vi "getStatusContainer.vi"(8 "error in (no error)":errorcluster, 11 "IComponent in":refnum<class "IComponent.lvclass">) -> (0 "error out":errorcluster, 2 "IComponentStatusContainer out":refnum<class "IComponentStatusContainer.lvclass">, 3 "IComponent out":refnum<class "IComponent.lvclass">)   [LabVIEW 2022 SP3, in "openDAQ.lvlib" / "IBaseObject.lvlib" / "IPropertyObject.lvlib" / "IComponent.lvlib" / "IComponent.lvclass"]
uses:
  <instrlib>/openDAQ/Public/Classes/IComponent/IComponent.lvclass
  C:/Program Files (x86)/National Instruments/LabVIEW 2022/instr.lib/openDAQ/Public/Classes/IBaseObject/IBaseObject.lvclass
  <instrlib>/openDAQ/Public/Classes/IComponentStatusContainer/IComponentStatusContainer.lvclass
  <instrlib>/openDAQ/Public/Classes/IBaseObject/IBaseObject.lvclass/IBaseObject.ctl
  <instrlib>/openDAQ/Public/Classes/IBaseObject/Accessor/Read reference.vi
  <instrlib>/openDAQ/Public/Classes/IBaseObject/Accessor/Write reference.vi
  <instrlib>/openDAQ/Binaries/Windows/x86/copendaq32.dll
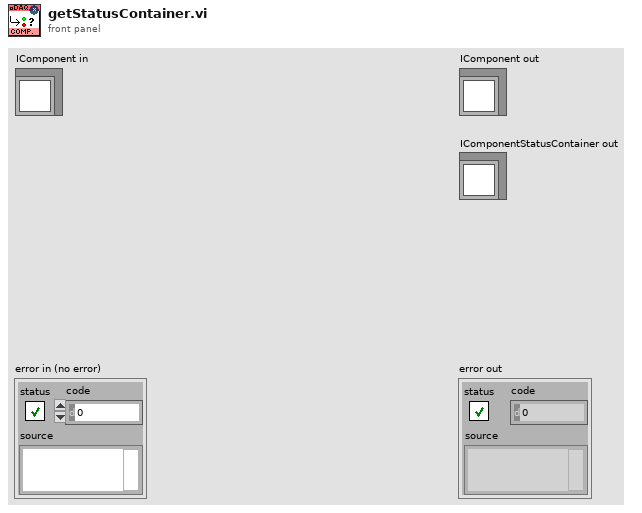
[diagram p1: front panel]
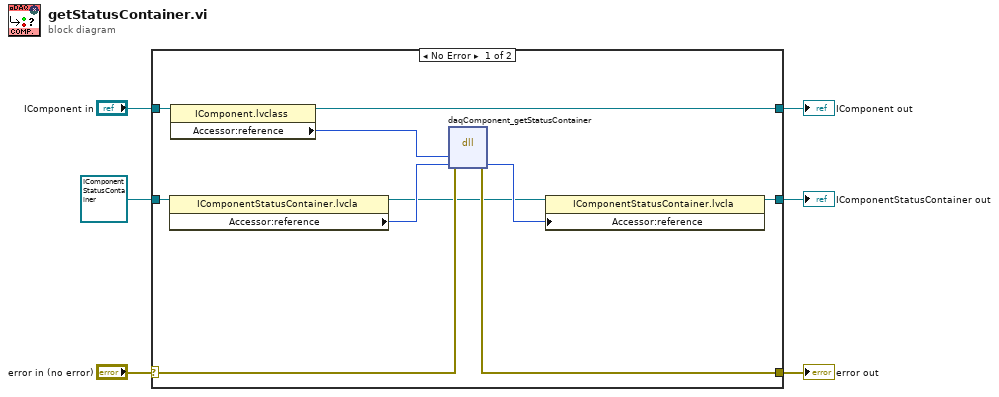
[diagram p0: block diagram]
diagram:
  n1 = case shown="No Error" "error in (no error)" {
    selector: "error in (no error)" -> [w11 w19]
    tunnel: [w14 w19] -> w5
    tunnel: [w12 w18] -> w3
    tunnel: "IComponent in" -> [w13 w18]
    tunnel: [w8 w17] -> w1
    tunnel: refnum<class "IComponentStatusContainer.lvclass"> refnum ("openDAQ.lvlib:IBaseObject.lvlib:ITag.lvlib:ITag.lvclass") -> [w7 w17]
    frame No Error {
      n2 = property class="IComponentStatusContainer.lvcla"(reference=w7) -> (reference out=w10:refnum<class "IComponentStatusContainer.lvclass">, "Accessor:reference"=w15:i64)  [unwired: 1 in, 1 out]
      n3 = property class="IComponent.lvclass"(reference=w13) -> (reference out=w12:refnum<class "IComponent.lvclass">, "Accessor:reference"=w9:i64)  [unwired: 1 in, 1 out]
      n4 = dll-call lib="C:/Program Files (x86)/National Instruments/LabVIEW 2022/instr.lib/openDAQ/Binaries/Windows/x86/copendaq*.*" fn="daqComponent_getStatusContainer"(error in=w11, "component"=w9, "statusContainer"=w15) -> (error out=w14:errorcluster, "statusContainer"=w16:i64)  [unwired: 4 in, 1 out]
      n5 = property class="IComponentStatusContainer.lvcla"(reference=w10, "Accessor:reference"=w16) -> (reference out=w8:refnum<class "IComponentStatusContainer.lvclass">)  [unwired: 1 in, 1 out]
    }
    frame Error {
    }
  }
  "error out" <- w5
  "IComponent out" <- w3
  "IComponentStatusContainer out" <- w1
